vi "未命名 13.vi"() -> ()   [LabVIEW 2016]
panel:
  out "周期设置 2":cluster{"启动":bool, "控制命令":T1}
  out "仪器最近一次启动时间":timestamp
  out "启动次数":i32
  in  "仪器运行状态":bool
  in  "周期设置":cluster{"启动":bool, "控制命令":T1}(xcontrol)
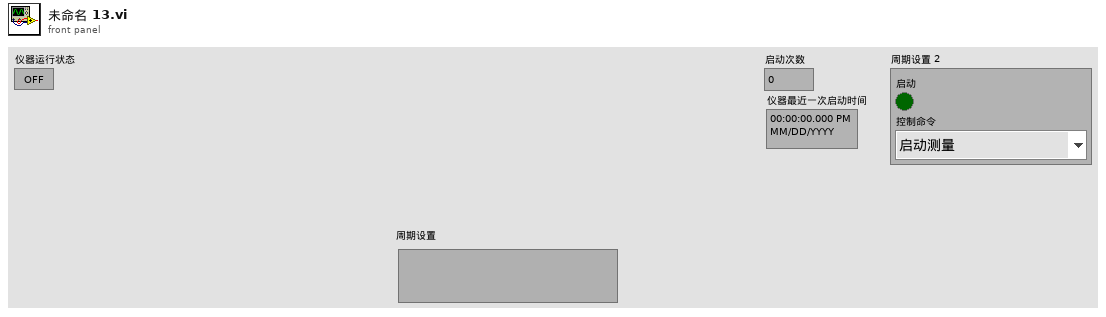
[diagram p1: front panel]
types:
  T1 = typedef "周期设置.xctl/国标控制命令.ctl" = enum16{"启动测量", "标样核查", "零点核查", "跨度核查", "空白测试", "平行样测试", "加标回收", "空白校准", "标样校准", "初始化（清洗）", "停止测试", "仪器重启", "校时", "模式设置", "测量间隔设置"}
  T2 = typedef "周期设置.xctl/周期模式设置.ctl" = enum16{"不启用", "定点模式", "间隔模式"}
  T3 = typedef "周期设置.xctl/定点周期设置.ctl" = cluster{"启动命令":T4, "启动命令 2":T4, "启动命令 3":T4, "启动命令 4":T4, "启动命令 5":T4, "启动命令 6":T4, "启动命令 7":T4, "启动命令 8":T4, "启动命令 9":T4, "启动命令 10":T4, "启动命令 11":T4, "启动命令 12":T4, "启动命令 13":T4, "启动命令 14":T4, "启动命令 15":T4, "启动命令 16":T4, "启动命令 17":T4, "启动命令 18":T4, "启动命令 19":T4, "启动命令 20":T4, "启动命令 21":T4, "启动命令 22":T4, "启动命令 23":T4, "启动命令 24":T4}
  T4 = typedef "周期设置.xctl/启动命令选择.ctl" = u16
  T5 = typedef "周期设置.xctl/间隔启动设置.ctl" = cluster{"启动命令":T4, "启动间隔":dbl, "启动次数":i32}
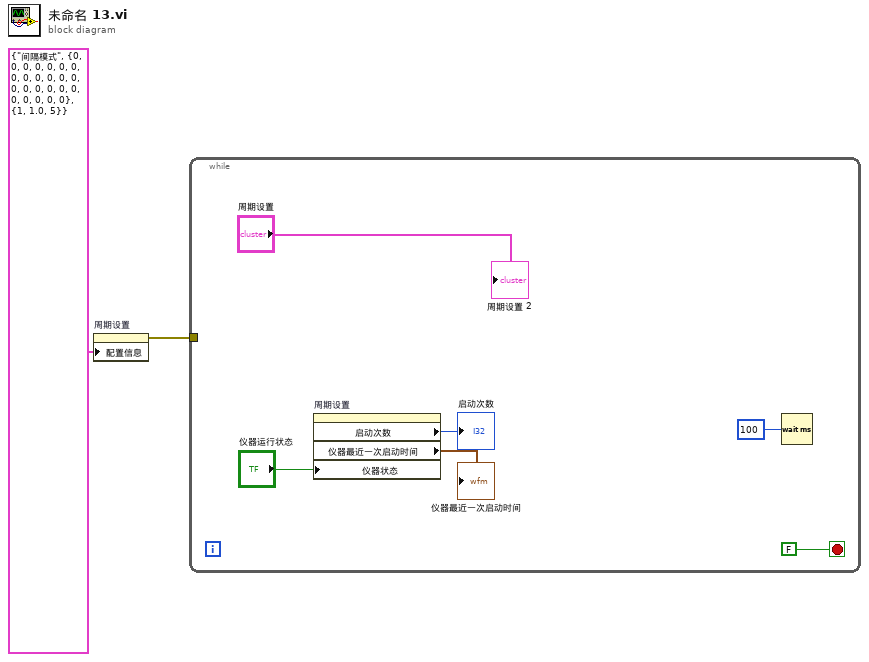
[diagram p0: block diagram]
diagram:
  n1 = property on="周期设置" class="周期设置 (严格)"("配置信息"=cluster{"周期模式":T2, "定点周期":T3, "间隔启动":T5} {"周期模式"=enum."间隔模式", "定点周期"={"启动命令"=0, "启动命令 2"=0, "启动命令 3"=0, "启动命令 4"=0, "启动命令 5"=0, "启动命令 6"=0, "启动命令 7"=0, "启动命令 8"=0, "启动命令 9"=0, "启动命令 10"=0, "启动命令 11"=0, "启动命令 12"=0, "启动命令 13"=0, "启动命令 14"=0, "启动命令 15"=0, "启动命令 16"=0, "启动命令 17"=0, "启动命令 18"=0, "启动命令 19"=0, "启动命令 20"=0, "启动命令 21"=0, "启动命令 22"=0, "启动命令 23"=0, "启动命令 24"=0}, "间隔启动"={"启动命令"=1, "启动间隔"=1.0, "启动次数"=5}}) -> (error out=w2:errorcluster)  [unwired: 2 in, 1 out]
  n2 = while {
    tunnel: w2 -> [_]
    stop <- FALSE stop-if-true
    n3 = property on="周期设置" class="周期设置 (严格)"("仪器状态"="仪器运行状态") -> ("启动次数"=→"启动次数":i32, "仪器最近一次启动时间"=→"仪器最近一次启动时间":timestamp)  [unwired: 2 in, 2 out]
    n4 = Wait (ms)(milliseconds to wait=u32 100 ("等待时间（毫秒）")) -> ()  [unwired: 1 out]
    "周期设置 2" <- "周期设置"
  }
